vi "make_current_structure_metajson.vi"(10 "structure_type":string="while", 11 "UID":i32) -> (3 "curr_while_metajson":string)   [LabVIEW 2020]
uses:
  <vilib>/JDP Science/JSONtext/support/Format JSON Array Text.vi
  <vilib>/JDP Science/JSONtext/support/Format JSON Object.vi
  <vilib>/JDP Science/JSONtext/JSONtext.lvlib
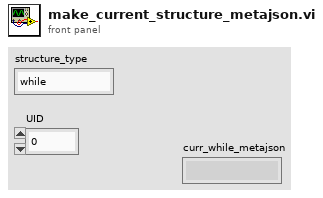
[diagram p1: front panel]
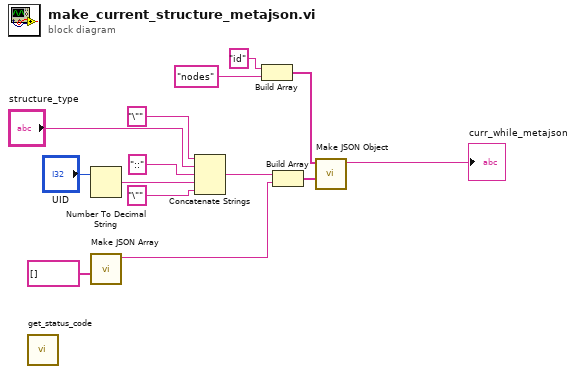
[diagram p0: block diagram]
diagram:
  n1 = call "get_status_code.vi"() -> ()  [unwired: 9 in, 2 out]
  n2 = Number To Decimal String(number="UID") -> (decimal integer string=w1:string)  [unwired: 1 in]
  n3 = call <vilib>:"Make JSON Array.vi"("JSON Elements"=string[] []) -> ("<JSON>"=w12:string)  [unwired: 9 in, 1 out]
  n4 = Concatenate Strings("\"" ("字符串"), "structure_type", "::" ("字符串"), w1, "\"" ("字符串")) -> (w14:string)
  n5 = Build Array("id" ("$Path or Item Name"), "nodes" ("元素")) -> (w8:string[])
  n6 = Build Array(w14, w12) -> (w9:string[])
  n7 = call <vilib>:"Make JSON Object.vi"("JSON Items"=w9, "Item Names"=w8) -> ("<JSON>"=→"curr_while_metajson":string)  [unwired: 8 in, 1 out]
